vi "FlatToRichcif_plugincore_PluginOverrides.vi"(5 "OutputClusterType":T1, 11 "InputCluster":T3) -> (3 "OutputCluster":T1)   [LabVIEW 2021, in "CIF_Manager_server.lvlib"]
uses:
  CIF_Manager_server.lvlib
  cif_plugincore_PluginOverrides_Flat.ctl
  cif_plugincore_TimingOverrides_Flat.ctl
  cif_plugincore_PluginOverrides.ctl
  cif_plugincore_TimingOverrides.ctl
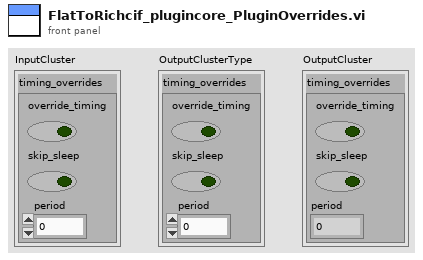
[diagram p1: front panel]
types:
  T1 = typedef "CIF_Manager_server.lvlib/cif_plugincore_PluginOverrides.ctl" = cluster{"timing_overrides":T2}
  T2 = typedef "CIF_Manager_server.lvlib/cif_plugincore_TimingOverrides.ctl" = cluster{"override_timing":bool, "skip_sleep":bool, "period":dbl}
  T3 = typedef "CIF_Manager_server.lvlib/cif_plugincore_PluginOverrides_Flat.ctl" = cluster{"timing_overrides":T4}
  T4 = typedef "CIF_Manager_server.lvlib/cif_plugincore_TimingOverrides_Flat.ctl" = cluster{"override_timing":bool, "skip_sleep":bool, "period":dbl}
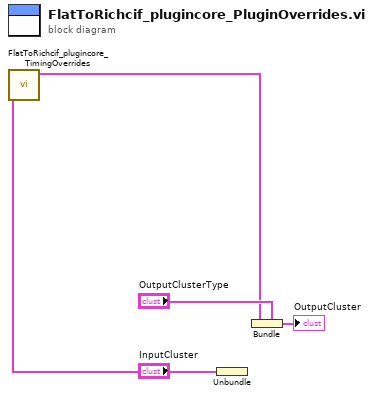
[diagram p0: block diagram]
diagram:
  n1 = Unbundle "Unbundle"("InputCluster") -> ("timing_overrides"=w2:T4)
  n2 = call "FlatToRichcif_plugincore_TimingOverrides.vi"("InputCluster"=w2) -> ("OutputCluster"=w1:T2)  [unwired: 10 in]
  n3 = Bundle "Bundle"(cluster="OutputClusterType", "timing_overrides"=w1) -> (→"OutputCluster":T1)
